vi "Seq Get Current Sequence.vi"(6 "config paths":T1, 8 "Error In":errorcluster, 9 "Segment Info In":T2, 10 "Basic Steps":string[](array[string]), 11 "VI Names":string[](array[string])) -> (0 "Error Out":errorcluster, 2 "Step Hisitory":string[](array[string]))   [LabVIEW 2018]
uses:
  type defs/Sequence Info.ctl
  type defs/config paths for seq def.ctl
panel:
  out "appended path":path
  out "file or folder exists?":bool
  out "File Name":string
  out "Add Step?":bool
  out "Segment Info Out":T2
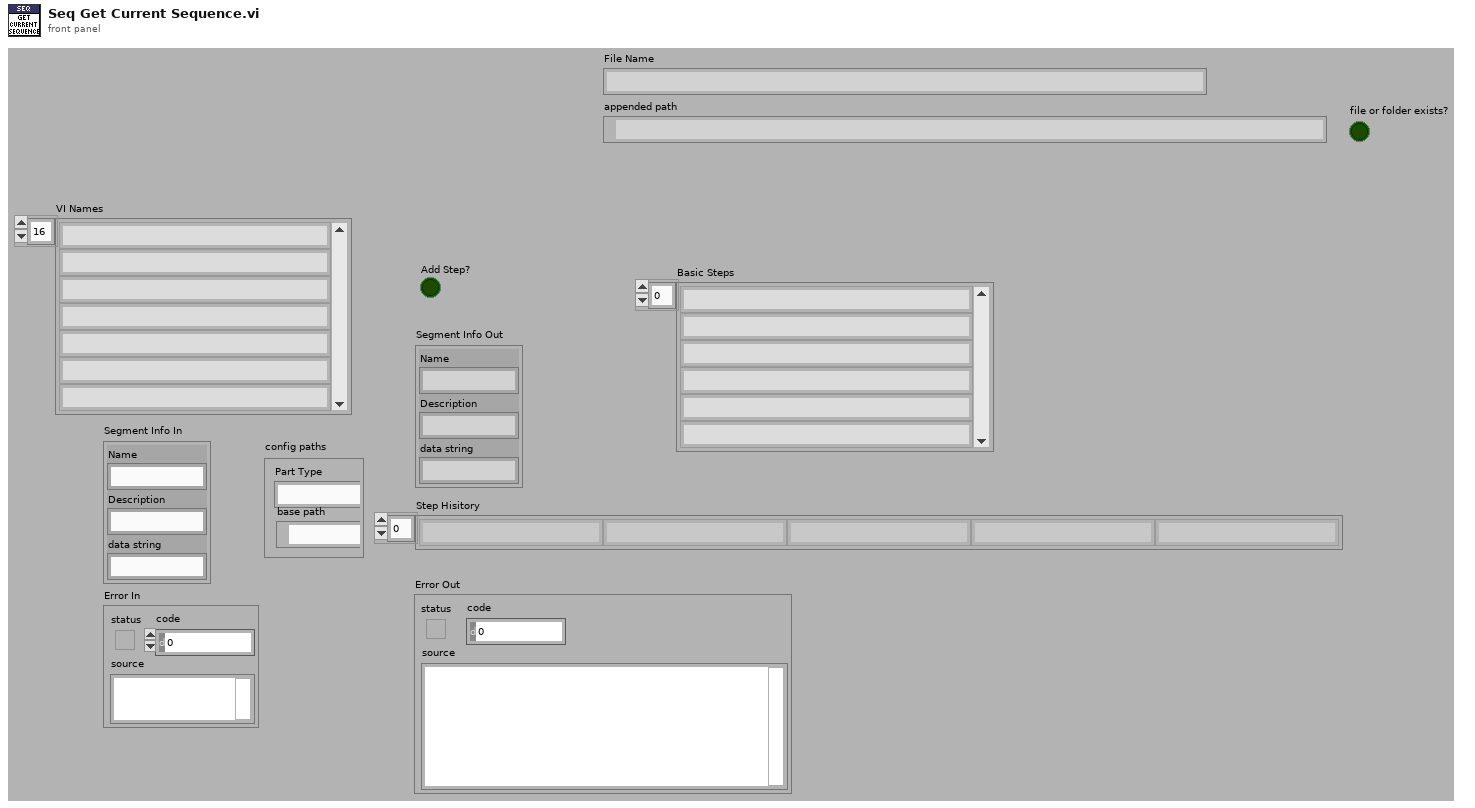
[diagram p1: front panel]
types:
  T1 = typedef "config paths for seq def.ctl" = cluster{"Part Type":string, "base path":path}
  T2 = typedef "Sequence Info.ctl" = cluster{"Name":string, "Description":string, "data string":string}
  T3 = enum32{"Bad", "Idle", "Run top level", "Running"}
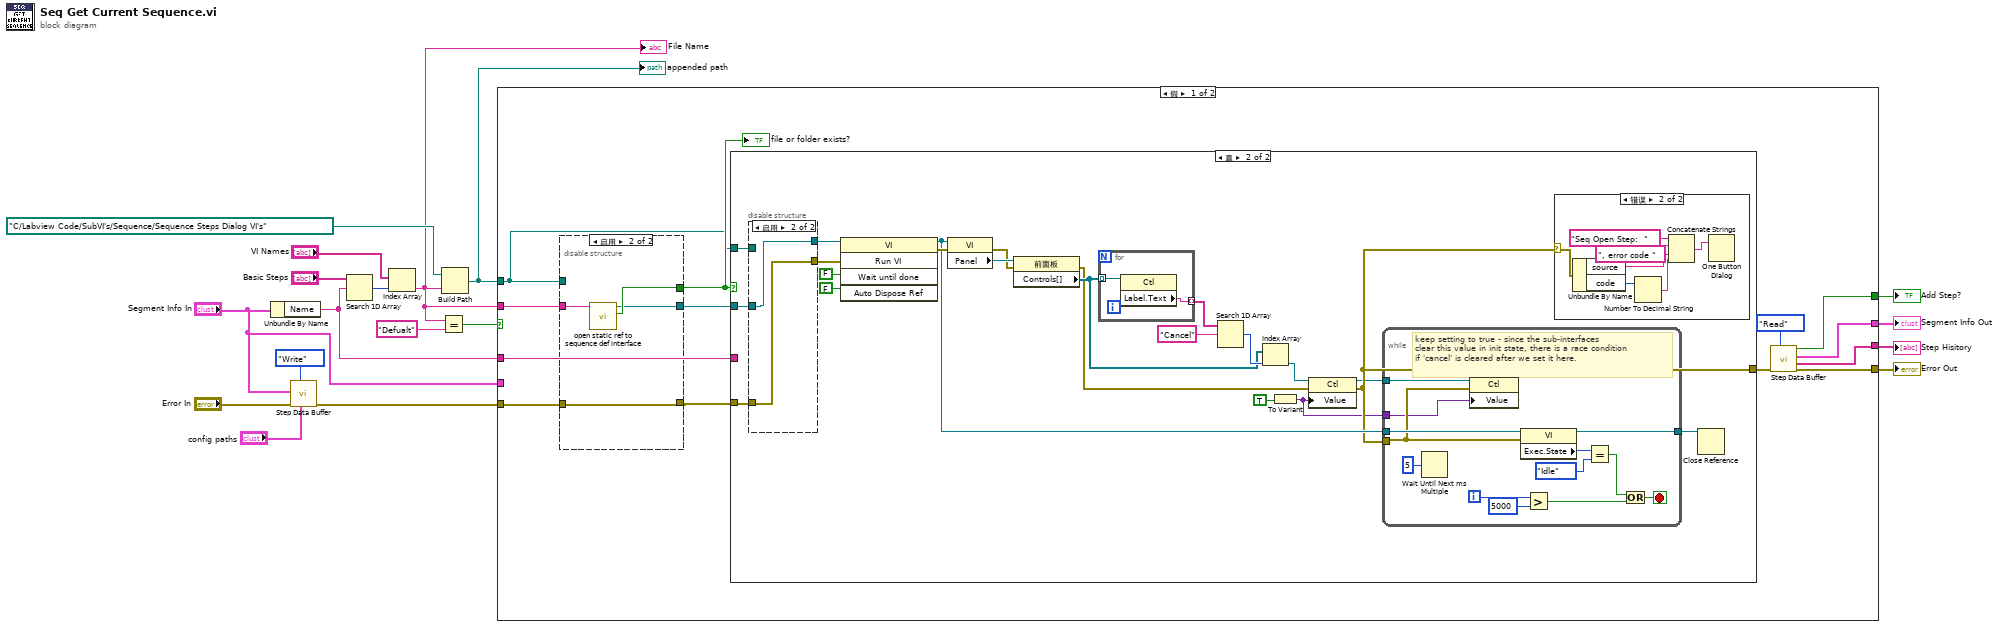
[diagram p0: block diagram]
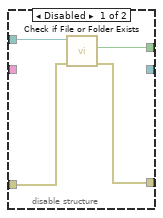
[diagram p2: hidden frame]
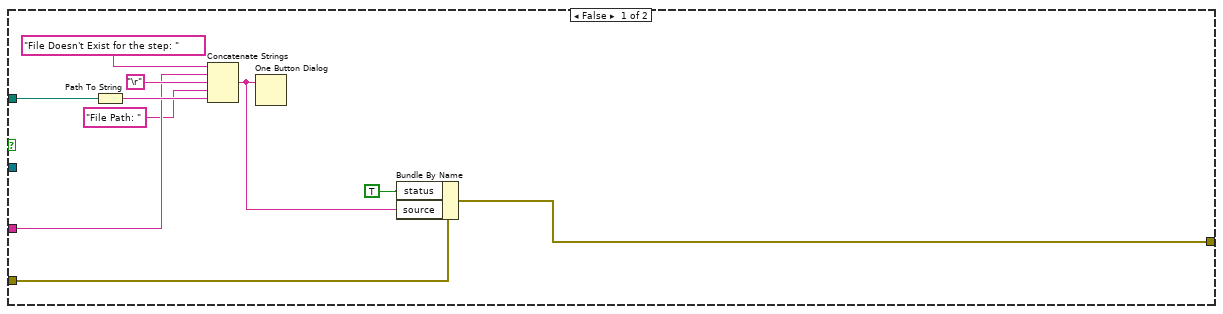
[diagram p3: hidden frame]
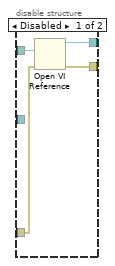
[diagram p4: hidden frame]
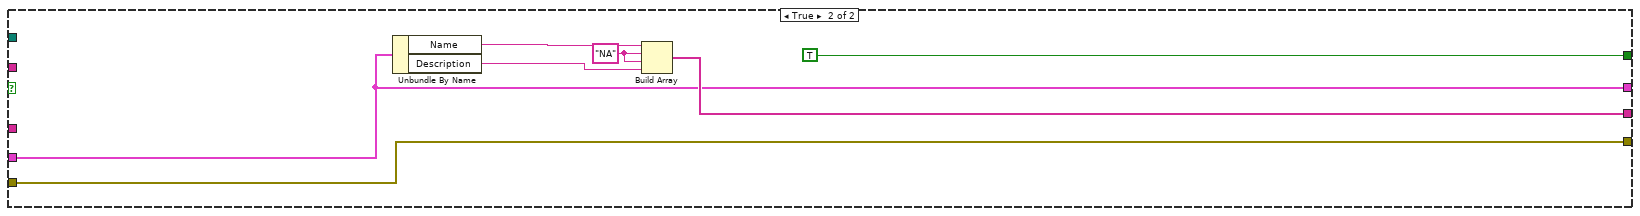
[diagram p6: hidden frame]
diagram:
  n1 = Unbundle By Name("Segment Info In") -> ("Name"=w13:string)
  n2 = call "Step Data Buffer.vi"("config paths"="config paths", "Mode"=enum16{"Init", "Read", "Write"}."Write", "Error In"="Error In", "Segment Data In"="Segment Info In") -> ("Error Out"=w10:errorcluster)  [unwired: 3 in, 4 out]
  n3 = Search 1D Array(1D array="Basic Steps", element=w13) -> (index of element=w9:i32)  [unwired: 1 in]
  n4 = Index Array(array="VI Names", index=w9) -> (element=w1:string)
  "File Name" <- w1
  n5 = Equal?(x=w1, y="Defualt") -> (x = y?=w7:bool)
  n6 = Build Path(base path=path "C:/Labview Code/SubVI's/Sequence/Sequence Steps Dialog VI's", name or relative path=w1) -> (appended path=w6:path)
  "appended path" <- w6
  n7 = case shown="假" w7 {
    tunnel: w6 -> [w30 _]
    tunnel: w10 -> [w29 w104]
    tunnel: [w25 w104] -> w14
    tunnel: w13 -> [w21 _]
    tunnel: [w24 w105] -> w18
    tunnel: [w22 TRUE ("Add Step?")] -> w5
    tunnel: "Segment Info In" -> [_ w102]
    tunnel: [w23 w102] -> w3
    tunnel: w1 -> [w20 _]
    frame False {
      n8 = disable-structure shown="启用" {
        disable-tunnel: [w35 w38] -> w31
        disable-tunnel: w30 -> [w34 _]
        disable-tunnel: w29 -> [w33 w37]
        disable-tunnel: [w32 w37] -> w28
        disable-tunnel: w20 -> [_ w39]
        disable-tunnel: [_ w36] -> w19
        frame Disabled {
          n9 = call <vilib>:"Check if File or Folder Exists.vi"("error in (no error)"=w33, "path"=w34) -> ("error out"=w32:errorcluster, "file or folder exists?"=w35:bool)  [unwired: 7 in, 1 out]
        }
        frame Enabled {
          n10 = call "open static ref to sequence def interface.vi"("vi name"=w39) -> ("exists"=w38:bool, "VI out"=w36:refnum<vi>)  [unwired: 9 in]
        }
      }
      "file or folder exists?" <- w31
      n11 = case shown="真" w31 {
        tunnel: w30 -> [w49 w71]
        tunnel: [w42 w57] -> w26
        tunnel: w28 -> [w43 w70]
        tunnel: w21 -> [w45 _]
        tunnel: w19 -> [_ w53]
        frame False {
          n12 = Path To String(path=w49) -> (string=w48:string)
          n13 = Concatenate Strings("File Doesn't Exist for the step: " ("string"), w45, "\r", "File Path: " ("string"), w48) -> (w41:string)
          n14 = One Button Dialog(message=w41) -> ()  [unwired: 1 in, 1 out]
          n15 = Bundle By Name(cluster=w43, "status"=TRUE, "source"=w41) -> (w42:errorcluster)
        }
        frame True {
          n16 = disable-structure shown="启用" {
            disable-tunnel: w71 -> [w72 _]
            disable-tunnel: w70 -> [w75 w77]
            disable-tunnel: [w74 w77] -> w55
            disable-tunnel: [w73 w76] -> w54
            disable-tunnel: w53 -> [_ w76]
            frame Disabled {
              n17 = Open VI Reference(vi path=w72, error in (no error)=w75) -> (vi reference=w73:refnum<vi>, error out=w74:errorcluster)  [unwired: 4 in]
            }
            frame Enabled {
            }
          }
          n18 = invoke class="VI" method="Run VI"(reference=w54, error in=w55, "Wait until done"=FALSE ("Wait Until Done"), "Auto Dispose Ref"=FALSE ("Auto Dispose Reference")) -> (reference out=w58:refnum<vi>, error out=w60:errorcluster)  [unwired: 1 in, 3 out]
          n19 = property class="VI"(reference=w58, error in=w60) -> (error out=w61:errorcluster, "Panel"=w68:refnum<vi>)  [unwired: 1 out]
          n20 = property class="前面板"(reference=w68, error in=w61) -> (error out=w52:errorcluster, "Controls[]"=w64:refnum<vi>[])  [unwired: 1 out]
          n21 = for {
            tunnel: w64 -> [w92] mode=indexing
            tunnel: [w91] -> w67 mode=indexing
            n22 = property class="Ctl"(reference=w92) -> ("Label.Text"=w91:string)  [unwired: 1 in, 2 out]
          }
          n23 = Search 1D Array(1D array=w67, element="Cancel") -> (index of element=w65:i32)  [unwired: 1 in]
          n24 = Index Array(array=w64, index=w65) -> (element=w63:refnum<vi>)
          n25 = To Variant(anything=TRUE) -> (Variant=w50:variant)
          n26 = property class="Ctl"(reference=w63, error in=w52, "Value"=w50) -> (reference out=w51:refnum<vi>, error out=w57:errorcluster)
          n27 = while {
            tunnel: w58 -> [w90]
            tunnel: w57 -> [w79]
            tunnel: [w82] -> w56
            tunnel: w51 -> [w81]
            tunnel: w50 -> [w78]
            i -> [w85]
            stop <- w87 stop-if-true
            # "keep setting to true - since the sub-interfaces\nclear this value in init state, there is a race condition\nif 'cancel' is cleared after we set it here."
            n28 = Wait Until Next ms Multiple(millisecond multiple=u32 5) -> ()  [unwired: 1 out]
            n29 = property class="Ctl"(reference=w81, error in=w79, "Value"=w78) -> ()  [unwired: 2 out]
            n30 = property class="VI"(reference=w90, error in=w79) -> (reference out=w82:refnum<vi>, "Exec.State"=w89:T3)  [unwired: 1 out]
            n31 = Greater?(x=w85, y=5000) -> (0:w83:bool)
            n32 = Equal?(x=w89, y=T3."Idle") -> (x = y?=w86:bool)
            n33 = Or(x=w86, y=w83) -> (x .or. y?=w87:bool)
          }
          n34 = case shown="错误" w57 {
            selector: w57 -> [_ w98]
            frame No Error {
            }
            frame Error {
              n35 = Unbundle By Name(w98) -> ("source"=w96:string, "code"=w94:i32)
              n36 = Number To Decimal String(number=w94) -> (decimal integer string=w93:string)  [unwired: 1 in]
              n37 = Concatenate Strings("Seq Open Step:  " ("message"), w96, ", error code " ("string"), w93) -> (w97:string)
              n38 = One Button Dialog(message=w97) -> ()  [unwired: 1 in, 1 out]
            }
          }
          n39 = Close Reference(reference=w56) -> ()  [unwired: 1 in, 1 out]
        }
      }
      n40 = call "Step Data Buffer.vi"("Mode"=enum16{"Init", "Read", "Write"}."Read", "Error In"=w26) -> ("Error Out"=w25:errorcluster, "Step Hisitory Out"=w24:string[], "Segment Data Out"=w23:T2, "Add Step? Out"=w22:bool)  [unwired: 5 in, 1 out]
    }
    frame True {
      w106 = "NA" ("element")
      n41 = Unbundle By Name(w102) -> ("Name"=w101:string, "Description"=w100:string)
      n42 = Build Array(w101, w106, w106, w100) -> (w105:string[])
    }
  }
  "Step Hisitory" <- w18
  "Segment Info Out" <- w3
  "Add Step?" <- w5
  "Error Out" <- w14
